vi "Go To XY.vi"(7 "Control Cluster":T1 {"Yaw Speed" scale=-1.0..1.0; "Vertical Speed" scale=-1.0..1.0; "Pitch" scale=-1.0..1.0; "Roll" scale=-1.0..1.0}, 8 "Y goal":dbl, 9 "X goal":dbl, 10 "Y current":dbl, 11 "X current":dbl) -> (3 "Control Cluster":T1)   [LabVIEW 2014]
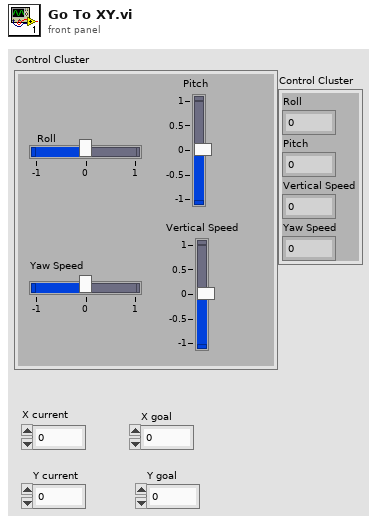
[diagram p1: front panel]
types:
  T1 = cluster{"Roll":sgl, "Pitch":sgl, "Vertical Speed":sgl, "Yaw Speed":sgl}
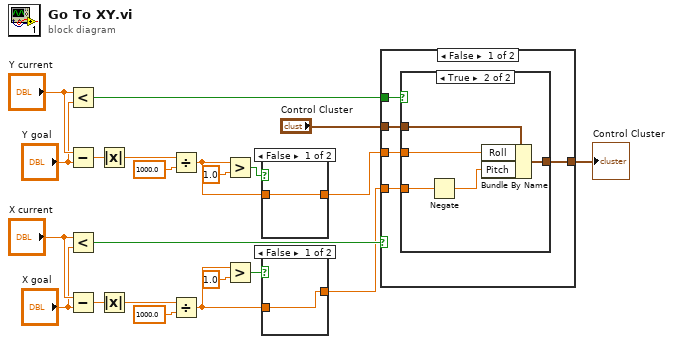
[diagram p0: block diagram]
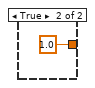
[diagram p2: hidden frame]
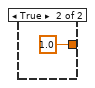
[diagram p3: hidden frame]
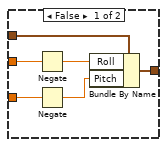
[diagram p4: hidden frame]
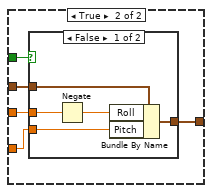
[diagram p5: hidden frame]
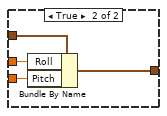
[diagram p6: hidden frame]
diagram:
  n1 = Less?(x="Y current", y="Y goal") -> (x < y?=w21:bool)
  n2 = Subtract(x="Y current", y="Y goal") -> (x-y=w10:dbl)
  n3 = Less?(x="X current", y="X goal") -> (x < y?=w22:bool)
  n4 = Subtract(x="X current", y="X goal") -> (x-y=w16:dbl)
  n5 = Absolute Value(x=w10) -> (abs(x)=w9:dbl)
  n6 = Absolute Value(x=w16) -> (abs(x)=w15:dbl)
  n7 = Divide(x=w9, y=1000.0) -> (x/y=w5:dbl)
  n8 = Divide(x=w15, y=1000.0) -> (x/y=w11:dbl)
  n9 = Greater?(x=w5, y=1.0) -> (0:w6:bool)
  n10 = Greater?(x=w11, y=1.0) -> (0:w12:bool)
  n11 = case shown="False" w6 {
    tunnel: w5 -> [w23 _]
    tunnel: [w23 1.0] -> w2
    frame False {
    }
    frame True {
    }
  }
  n12 = case shown="False" w12 {
    tunnel: w11 -> [w25 _]
    tunnel: [w25 1.0] -> w1
    frame False {
    }
    frame True {
    }
  }
  n13 = case shown="False" w22 {
    tunnel: w21 -> [w29 w47]
    tunnel: "Control Cluster" -> [w31 w46]
    tunnel: [w30 w45] -> w19
    tunnel: w2 -> [w27 w44]
    tunnel: w1 -> [w28 w43]
    frame False {
      n14 = case shown="True" w29 {
        tunnel: w31 -> [w37 w42]
        tunnel: [w36 w41] -> w30
        tunnel: w28 -> [w33 w38]
        tunnel: w27 -> [w32 w39]
        frame False {
          n15 = Negate(x=w32) -> (-x=w35:dbl)
          n16 = Negate(x=w33) -> (-x=w34:dbl)
          n17 = Bundle By Name(cluster=w37, "Roll"=w35, "Pitch"=w34) -> (w36:T1)
        }
        frame True {
          n18 = Negate(x=w38) -> (-x=w40:dbl)
          n19 = Bundle By Name(cluster=w42, "Roll"=w39, "Pitch"=w40) -> (w41:T1)
        }
      }
    }
    frame True {
      n20 = case shown="False" w47 {
        tunnel: w46 -> [w52 w56]
        tunnel: [w51 w55] -> w45
        tunnel: w44 -> [w48 w54]
        tunnel: w43 -> [w50 w53]
        frame False {
          n21 = Negate(x=w48) -> (-x=w49:dbl)
          n22 = Bundle By Name(cluster=w52, "Roll"=w49, "Pitch"=w50) -> (w51:T1)
        }
        frame True {
          n23 = Bundle By Name(cluster=w56, "Roll"=w54, "Pitch"=w53) -> (w55:T1)
        }
      }
    }
  }
  "Control Cluster" <- w19
